vi "Run Time Value Unit to Register Data.vi"(0 "Run Time Value":dbl=1.0 caption="运行时间值" min=0.001, 3 "Run Time Unit":u16(ring)=1 caption="运行时间单位" items=["h", "min", "s"]) -> (7 "Valid Result":bool caption="有效结果？", 9 "Value Reg Data":dbl caption="值寄存器", 10 "Unit Reg Data":dbl caption="单位寄存器")   [LabVIEW 2023, in "Longer Pump dLSP501 Series.lvlib"]
uses:
  <instrlib>/Longer Pump dLSP501 Modbus RTU Series/Longer Pump dLSP501 Series.lvlib
panel:
  out "已强制转换(x)":dbl caption="强制转换结果"
  out "范围内？":bool caption="范围内 ?"
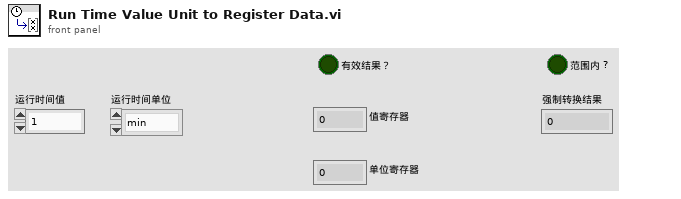
[diagram p1: front panel]
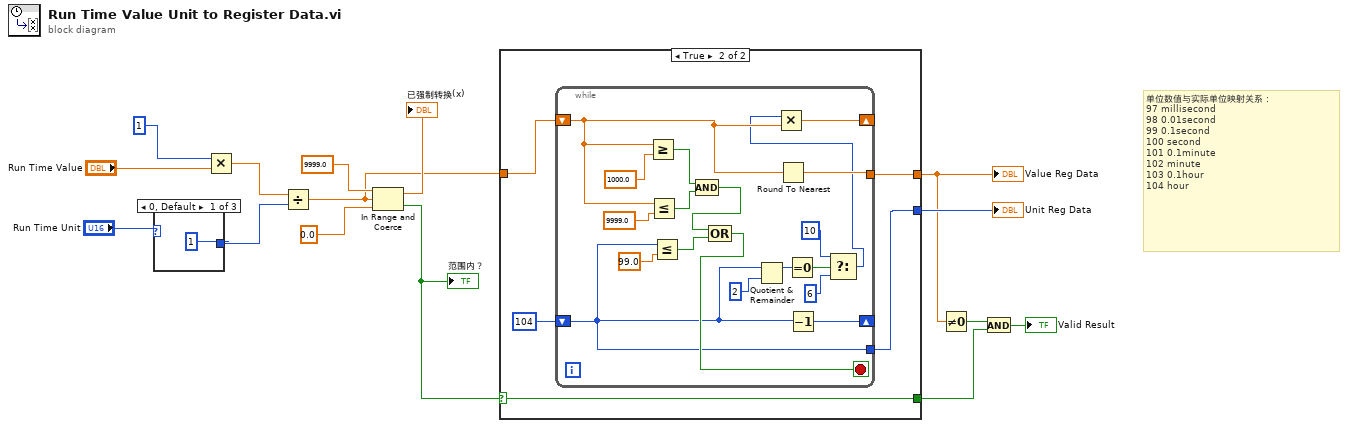
[diagram p0: block diagram]
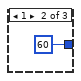
[diagram p2: hidden frame]
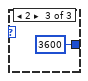
[diagram p3: hidden frame]
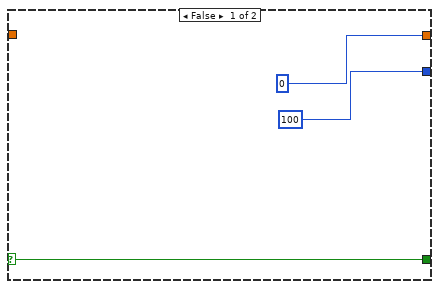
[diagram p4: hidden frame]
diagram:
  # "单位数值与实际单位映射关系：\n97\tmillisecond\n98\t0.01second\n99\t0.1second\n100\tsecond\n101\t0.1minute\n102\tminute\n103\t0.1hour\n104\thour"
  n1 = case shown="0, Default" "Run Time Unit" {
    tunnel: [1 60 3600] -> w8
    frame 0, Default {
    }
    frame 1 {
    }
    frame 2 {
    }
  }
  n2 = Multiply(x=u16 1 ("y"), y="Run Time Value") -> (x*y=w15:dbl)
  n3 = Divide(x=w15, y=w8) -> (x/y=w11:dbl)
  n4 = In Range and Coerce(upper limit=9999.0 ("x"), x=w11, lower limit=0.0 ("x")) -> (coerced(x)=→"已强制转换(x)":dbl, In Range?=w5:bool)
  "范围内？" <- w5
  n5 = case shown="True" w5 {
    selector: w5 -> [w21 w26]
    tunnel: w11 -> [_ w25]
    tunnel: [w21 w26] -> w2
    tunnel: [100 w22] -> w10
    tunnel: [0 w23] -> w3
    frame False {
    }
    frame True {
      n6 = while {
        shift-right: [w45] -> _
        shift-left: w25 -> [w34]
        shift-right: [w37] -> _
        shift-left: 104 -> [w33]
        tunnel: [w35] -> w23
        tunnel: [w33] -> w22
        stop <- w39 stop-if-true
        n7 = Greater Or Equal?(x=w34, y=1000.0 ("x")) -> (x >= y?=w42:bool)
        n8 = Less Or Equal?(x=w34, y=9999.0 ("x")) -> (x <= y?=w41:bool)
        n9 = Less Or Equal?(x=w33, y=99.0 ("x")) -> (x <= y?=w36:bool)
        n10 = Compound Arithmetic op=AND ("复合运算")(w42, w41) -> (w40:bool)
        n11 = Compound Arithmetic op=OR ("复合运算")(w40, w36) -> (w39:bool)
        n12 = Quotient & Remainder(x=w33, y=2) -> (x-y*floor(x/y)=w31:i32)  [unwired: 1 out]
        n13 = Round To Nearest(number=w34) -> (nearest integer value=w35:dbl)
        n14 = Equal To 0?(x=w31) -> (x = 0?=w30:bool)
        n15 = Decrement(x=w33) -> (x-1=w37:i32)
        n16 = Select(t=10, s=w30, f=6) -> (s? t:f=w27:i32)
        n17 = Multiply(x=w27, y=w34) -> (x*y=w45:dbl)
      }
    }
  }
  "Value Reg Data" <- w3
  "Unit Reg Data" <- w10
  n18 = Not Equal To 0?(x=w3) -> (x != 0?=w4:bool)
  n19 = And(x=w4, y=w2) -> (x .and. y?=→"Valid Result":bool)
